vi "Convert HEX to Raw.vi"(4 "Raw Data Flattened to String":string) -> (1 "Raw Flattened String":string)   [LabVIEW 2023]
panel:
  out "length":i32
  out "length":i32
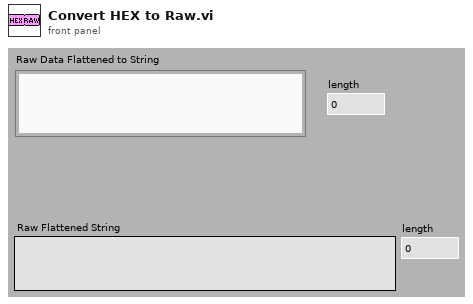
[diagram p1: front panel]
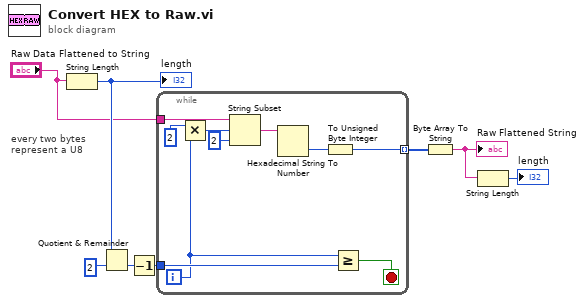
[diagram p0: block diagram]
diagram:
  # "every two bytes represent a U8"
  n1 = String Length(string="Raw Data Flattened to String") -> (length=w5:i32)
  "length" <- w5
  n2 = Quotient & Remainder(x=w5, y=2 ("length (rest)")) -> (floor(x/y)=w4:i32)  [unwired: 1 out]
  n3 = Decrement(x=w4) -> (x-1=w1:i32)
  n4 = while {
    tunnel: [w9] -> w8 mode=indexing
    tunnel: "Raw Data Flattened to String" -> [w18]
    tunnel: w1 -> [w11]
    i -> [w10]
    stop <- w12 stop-if-true
    n5 = Multiply(x=2 ("length (rest)"), y=w10) -> (x*y=w14:i32)
    n6 = String Subset(string=w18, offset (0)=w14, length (rest)=2 ("length (rest)")) -> (substring=w17:string)
    n7 = Hexadecimal String To Number(string=w17) -> (number=w16:u32)  [unwired: 2 in, 1 out]
    n8 = To Unsigned Byte Integer(number=w16) -> (unsigned 8bit integer=w9:u8)
    n9 = Greater Or Equal?(x=w10, y=w11) -> (x >= y?=w12:bool)
  }
  n10 = Byte Array To String(unsigned byte array=w8) -> (string=w2:string)
  "Raw Flattened String" <- w2
  n11 = String Length(string=w2) -> (length=→"length":i32)
